vi "Get Progress Queue.vi"(8 "error in":errorcluster, 11 "Enable Tracking?":bool=TRUE) -> (0 "error out":errorcluster, 3 "Progress queue":T1)   [LabVIEW 2019, in "Project.Dependencies Finder.lvlib"]
uses:
  Project.Dependencies Finder.lvlib
  Ctl/Ctl_Progress Queue.ctl
  Private/Gobal_Progress Tracking State.vi
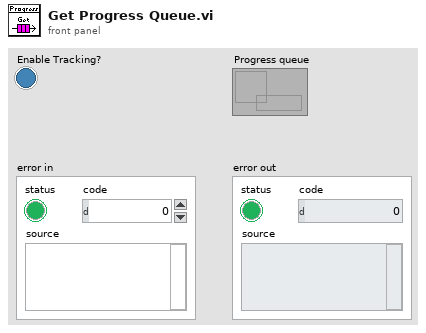
[diagram p1: front panel]
types:
  T1 = typedef "Project.Dependencies Finder.lvlib/Ctl_Progress Queue.ctl" = refnum<queue>
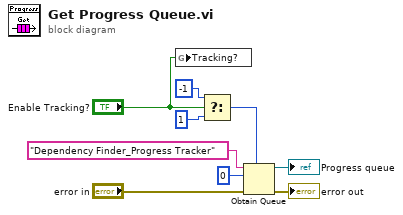
[diagram p0: block diagram]
diagram:
  n1 = global write "Gobal_Progress Tracking State.vi" "Tracking?"("Enable Tracking?") -> ()
  n2 = Select(t=-1 ("max queue size (-1, unlimited)"), s="Enable Tracking?", f=1 ("max queue size (-1, unlimited)")) -> (s? t:f=w3:i32)
  n3 = Obtain Queue(max queue size (-1, unlimited)=w3, name (unnamed)="Dependency Finder_Progress Tracker" ("string"), element data type=0, error in (no error)="error in") -> (queue out=→"Progress queue":refnum<queue>, error out=→"error out":errorcluster)  [unwired: 1 in, 1 out]
